vi "Real Matrix to Compact Array.vi"(2 "matrix type":i32(ring) items=["lower triangular", "upper triangular", "symmetric matrix"], 3 "Matrix A":T1) -> (0 "error":i32, 1 "Compact Array":cluster{"Compact Array":dbl[], "array type":i32} {"array type" items=["lower triangular", "upper triangular", "symmetric matrix"]; "Compact Array" format="%.2f"})   [LabVIEW 2017, in "NI_AALBase.lvlib"]
uses:
  NI_AALBase.lvlib
  RealMatrix.ctl
  lvanlys.dll
  NI_Matrix.lvlib
panel:
  # "Real Matrix to Compact Array"
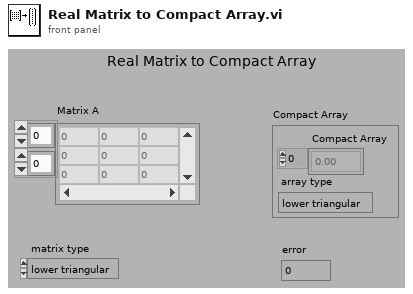
[diagram p1: front panel]
types:
  T1 = typedef "NI_Matrix.lvlib/RealMatrix.ctl" = dbl[][]
  T2 = cluster{"Compact Array":dbl[], "matrix type":i32}
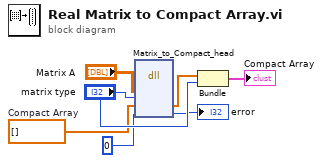
[diagram p0: block diagram]
diagram:
  w5 = dbl[] []  # Compact Array
  n1 = dll-call lib="C:/Program Files/National Instruments/LabVIEW 2017/resource/lvanlys.*" fn="Matrix_to_Compact_head"("Matrix A"="Matrix A", "matrix type"="matrix type", "Compact Array"=w5, 0) -> ("Compact Array"=w2:dbl[], →"error":i32)  [unwired: 6 in, 2 out]
  n2 = Bundle("Compact Array"=w2, "matrix type"="matrix type") -> (→"Compact Array":T2)  [unwired: 1 in]
